vi "NMEA_ParseMessage-GPRMC.vi"(9 "Error In":errorcluster, 10 "$GPRMC-message_IN":string) -> (1 "Error Out":errorcluster, 2 "$GPRMC-message_OUT":T1={"TimeStamp"=timestamp(0 s since 1904-01-01), "Validity"=FALSE, "Latitude"=0.0, "Latitude-Direction"=enum."North", "Longitude"=0.0, "Longitude-Direction"=enum."East", "Speed in knots"=0.0, "True course"=0.0, "Date Stamp"=timestamp(0 s since 1904-01-01), "Magnetic Variation (East/West)"=0.0} {"Magnetic Variation (East/West)" format="%.02f [deg]"; "Date Stamp" format="%<%x>T"; "True course" format="%.02f [deg]"; "Speed in knots" format="%.02f [kts]"; "Longitude" format="%0.4f [long]"; "Latitude" format="%.04f [lat]"; "TimeStamp" format="%<%.2X>T"})   [LabVIEW 2020, in "NMEA.lvlib"]
doc: "<B>GPRMC</B>\nRecommended minimum specific GPS/Transit data"
uses:
  NMEA.lvlib
  NMEA_GPRMC-data.ctl
  NMEA_LatitudeDirection.ctl
  NMEA_LongitudeDirection.ctl
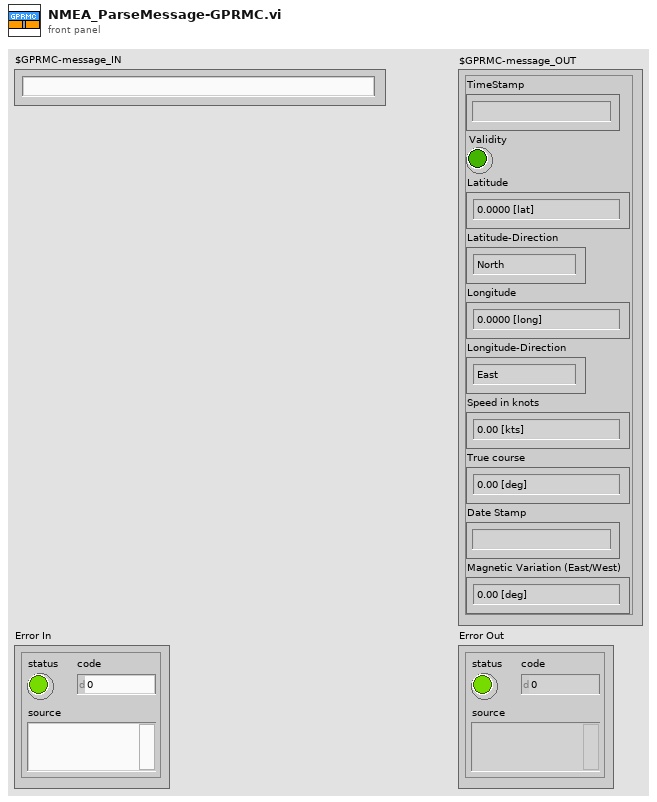
[diagram p1: front panel]
types:
  T1 = typedef "NMEA.lvlib/NMEA_GPRMC-data.ctl" = cluster{"TimeStamp":timestamp, "Validity":bool, "Latitude":dbl, "Latitude-Direction":T2, "Longitude":dbl, "Longitude-Direction":T3, "Speed in knots":dbl, "True course":dbl, "Date Stamp":timestamp, "Magnetic Variation (East/West)":dbl}
  T2 = typedef "NMEA.lvlib/NMEA_LatitudeDirection.ctl" = enum16{"", "North", "South"}
  T3 = typedef "NMEA.lvlib/NMEA_LongitudeDirection.ctl" = enum16{"", "East", "West"}
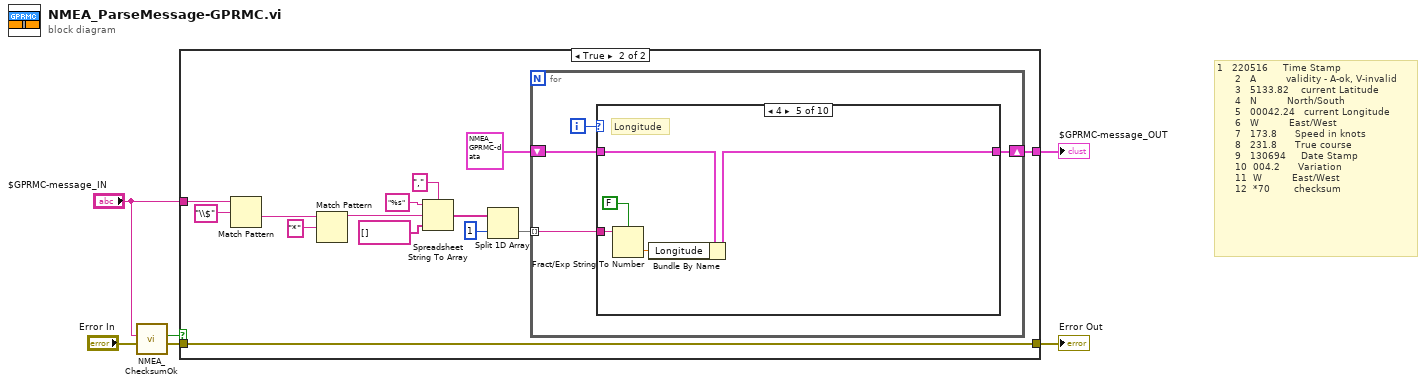
[diagram p0: block diagram]
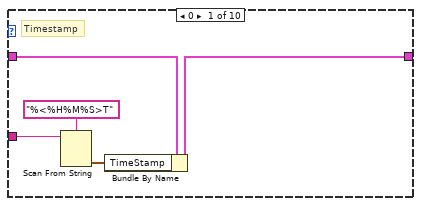
[diagram p3: hidden frame]
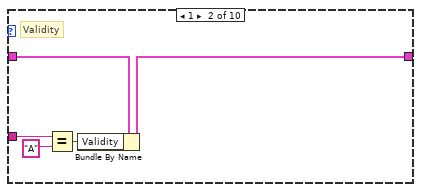
[diagram p4: hidden frame]
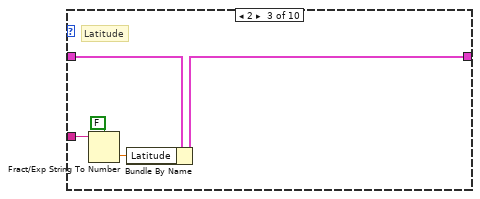
[diagram p5: hidden frame]
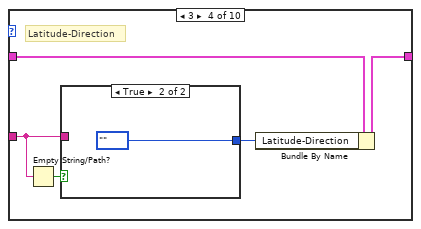
[diagram p6: hidden frame]
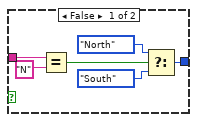
[diagram p7: hidden frame]
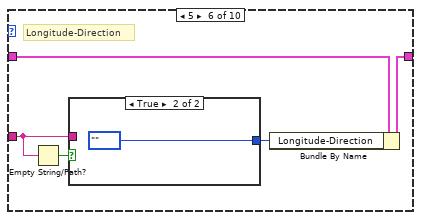
[diagram p8: hidden frame]
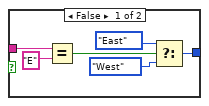
[diagram p9: hidden frame]
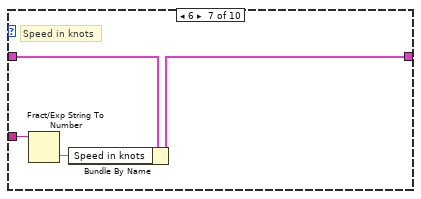
[diagram p10: hidden frame]
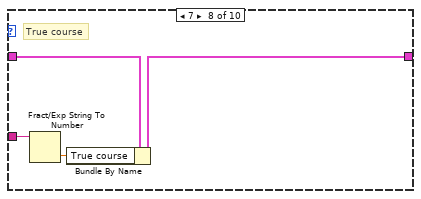
[diagram p11: hidden frame]
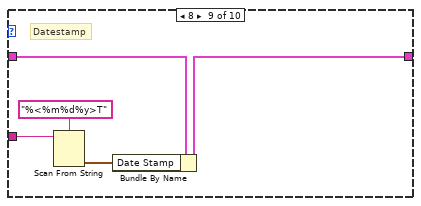
[diagram p12: hidden frame]
diagram:
  # "1   220516     Time Stamp\n      2   A          validity - A-ok, V-invalid\n      3   5133.82    current Latitude\n      4   N          North/South\n      5   00042.24   current Longitude\n      6   W          East/West\n      7   173.8      Speed in knots\n      8   231.8      True course\n      9   130694     Date Stamp\n      10  004.2      Variation\n      11  W          East/West\n      12  *70        checksum"
  n1 = call "NMEA_ChecksumOk.vi"("Error In"="Error In", "Sentence"="$GPRMC-message_IN") -> ("Error Out"=w1:errorcluster, "CheckSumOk?"=w4:bool)  [unwired: 8 in]
  n2 = case shown="True" w4 {
    tunnel: [_ w16] -> w6
    tunnel: "$GPRMC-message_IN" -> [_ w14]
    tunnel: w1 -> [w7 w9]
    tunnel: [w7 w9] -> w3
    frame False {
    }
    frame True {
      n3 = Match Pattern(string=w14, regular expression="\\$") -> (after substring=w13:string)  [unwired: 1 in, 3 out]
      n4 = Match Pattern(string=w13, regular expression="*") -> (before substring=w20:string)  [unwired: 1 in, 3 out]
      n5 = Spreadsheet String To Array(delimiter (Tab)=",", format string="%s", spreadsheet string=w20, array type (2D Dbl)=string[] []) -> (array=w11:string[])
      n6 = Split 1D Array(array=w11, index=1) -> (second subarray=w12:string[])  [unwired: 1 out]
      n7 = for {
        tunnel: w12 -> [w22] mode=indexing
        shift-right: [w24] -> w16
        shift-left: T1 {"TimeStamp"=timestamp(0 s since 1904-01-01), "Validity"=FALSE, "Latitude"=0.0, "Latitude-Direction"=enum."North", "Longitude"=0.0, "Longitude-Direction"=enum."East", "Speed in knots"=0.0, "True course"=0.0, "Date Stamp"=timestamp(0 s since 1904-01-01), "Magnetic Variation (East/West)"=0.0} ("$GPRMC-message_OUT") -> [w25]
        i -> [w23]
        n8 = case shown="4" w23 {
          tunnel: w25 -> [w30 w35 w40 w45 w57 w62 w73 w77 w82 w83]
          tunnel: [w29 w34 w39 w44 w56 w61 w72 w76 w81 w83] -> w24
          tunnel: w22 -> [w27 w33 w38 w42 w55 w59 w71 w75 w79 _]
          frame 0 {
            # "Timestamp"
            n9 = Scan From String(format string="%<%H%M%S>T", input string=w27) -> (output 1=w26:timestamp)  [unwired: 3 in, 3 out]
            n10 = Bundle By Name(cluster=w30, "TimeStamp"=w26) -> (w29:T1)
          }
          frame 1 {
            # "Validity"
            n11 = Equal?(x=w33, y="A") -> (x = y?=w31:bool)
            n12 = Bundle By Name(cluster=w35, "Validity"=w31) -> (w34:T1)
          }
          frame 2 {
            # "Latitude"
            n13 = Fract/Exp String To Number(use system decimal point (T)=FALSE, string=w38) -> (number=w37:dbl)  [unwired: 2 in, 1 out]
            n14 = Bundle By Name(cluster=w40, "Latitude"=w37) -> (w39:T1)
          }
          frame 3 {
            # "Latitude-Direction"
            n15 = Empty String/Path?(string/path=w42) -> (empty?=w41:bool)
            n16 = case shown="True" w41 {
              tunnel: [w48 NMEA_LatitudeDirection."" ("f")] -> w43
              tunnel: w42 -> [w46 _]
              frame False {
                n17 = Equal?(x=w46, y="N") -> (x = y?=w50:bool)
                n18 = Select(t=NMEA_LatitudeDirection."North" ("Latitude-Direction"), s=w50, f=NMEA_LatitudeDirection."South") -> (s? t:f=w48:T2)
              }
              frame True {
              }
            }
            n19 = Bundle By Name(cluster=w45, "Latitude-Direction"=w43) -> (w44:T1)
          }
          frame 4 {
            # "Longitude"
            n20 = Fract/Exp String To Number(use system decimal point (T)=FALSE, string=w55) -> (number=w54:dbl)  [unwired: 2 in, 1 out]
            n21 = Bundle By Name(cluster=w57, "Longitude"=w54) -> (w56:T1)
          }
          frame 5 {
            # "Longitude-Direction"
            n22 = Empty String/Path?(string/path=w59) -> (empty?=w58:bool)
            n23 = case shown="True" w58 {
              tunnel: w59 -> [w68 _]
              tunnel: [w64 NMEA_LongitudeDirection."" ("f")] -> w60
              frame False {
                n24 = Equal?(x=w68, y="E") -> (x = y?=w66:bool)
                n25 = Select(t=NMEA_LongitudeDirection."East" ("Longitude-Direction"), s=w66, f=NMEA_LongitudeDirection."West") -> (s? t:f=w64:T3)
              }
              frame True {
              }
            }
            n26 = Bundle By Name(cluster=w62, "Longitude-Direction"=w60) -> (w61:T1)
          }
          frame 6 {
            # "Speed in knots"
            n27 = Fract/Exp String To Number(string=w71) -> (number=w70:dbl)  [unwired: 3 in, 1 out]
            n28 = Bundle By Name(cluster=w73, "Speed in knots"=w70) -> (w72:T1)
          }
          frame 7 {
            # "True course"
            n29 = Fract/Exp String To Number(string=w75) -> (number=w74:dbl)  [unwired: 3 in, 1 out]
            n30 = Bundle By Name(cluster=w77, "True course"=w74) -> (w76:T1)
          }
          frame 8 {
            # "Datestamp"
            n31 = Scan From String(format string="%<%m%d%y>T", input string=w79) -> (output 1=w78:timestamp)  [unwired: 3 in, 3 out]
            n32 = Bundle By Name(cluster=w82, "Date Stamp"=w78) -> (w81:T1)
          }
          frame Default {
          }
        }
      }
    }
  }
  "$GPRMC-message_OUT" <- w6
  "Error Out" <- w3
